vi "CHOP_IN.vi"(5 "IN VARIANT":variant, 7 "Ip":string, 9 "Name in":string, 11 "error in (no error)":errorcluster) -> (6 "OUT VARIANT":variant, 10 "Valid data":bool, 15 "error out":errorcluster)   [LabVIEW 2015]
uses:
  CHOPS_COUPLE_separator_string.ctl
panel:
  out "right":string
  out "Left":string
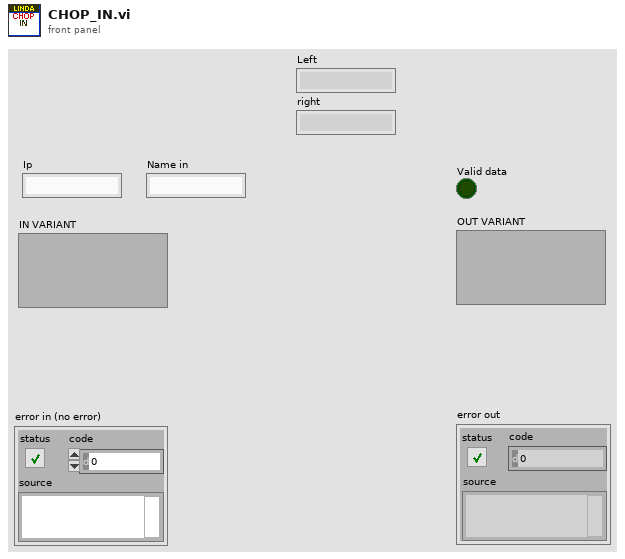
[diagram p1: front panel]
types:
  T1 = typedef "CHOPS_COUPLE_separator_string.ctl" = string
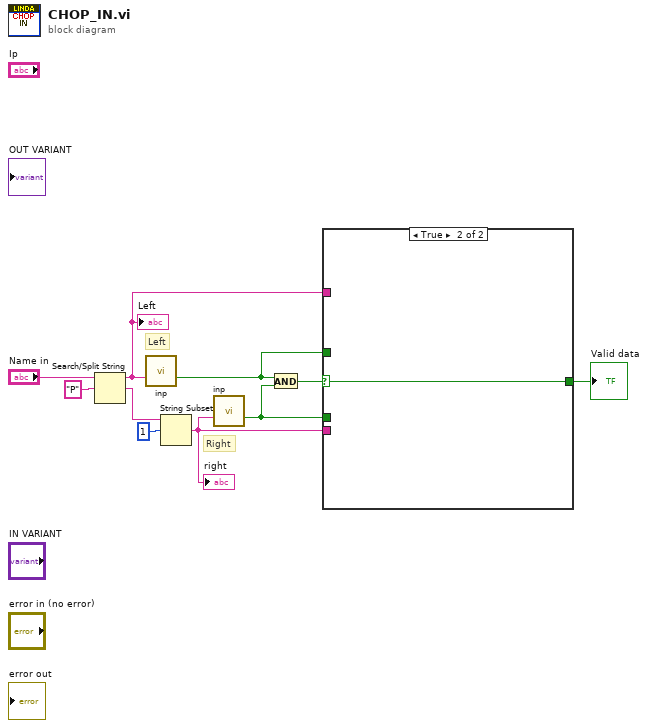
[diagram p0: block diagram]
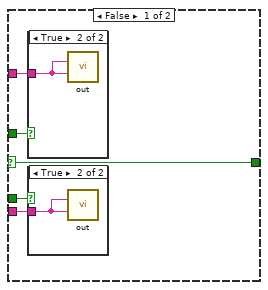
[diagram p2: hidden frame]
diagram:
  # "Right"
  # "Left"
  n1 = Search/Split String(string="Name in", search string/char (-)=T1 "P") -> (substring before match=w6:string, match + rest of string=w9:string)  [unwired: 1 in, 1 out]
  "Left" <- w6
  n2 = call "inp.vi"("Name in"=w6) -> ("Valid data"=w3:bool)  [unwired: 12 in, 2 out]
  n3 = String Subset(string=w9, offset (0)=1) -> (substring=w5:string)  [unwired: 1 in]
  "right" <- w5
  n4 = call "inp.vi"("Name in"=w5) -> ("Valid data"=w4:bool)  [unwired: 12 in, 2 out]
  n5 = And(x=w3, y=w4) -> (x .and. y?=w7:bool)
  n6 = case shown="True" w7 {
    selector: w7 -> [w11 w18]
    tunnel: w6 -> [w15 _]
    tunnel: w3 -> [w12 _]
    tunnel: w5 -> [w14 _]
    tunnel: w4 -> [w13 _]
    tunnel: [w11 w18] -> w2
    frame False {
      n7 = case shown="True" w12 {
        tunnel: w15 -> [_ w17]
        frame False {
        }
        frame True {
          n8 = call "out.vi"("IN VARIANT"=w17, "Name in"=w17) -> ()  [unwired: 12 in, 2 out]
        }
      }
      n9 = case shown="True" w13 {
        tunnel: w14 -> [_ w16]
        frame False {
        }
        frame True {
          n10 = call "out.vi"("IN VARIANT"=w16, "Name in"=w16) -> ()  [unwired: 12 in, 2 out]
        }
      }
    }
    frame True {
    }
  }
  "Valid data" <- w2
